vi "Time.vi"() -> ()   [LabVIEW 2025]
panel:
  out "date/time string":string
  out "Waveform Chart":dbl(graph)
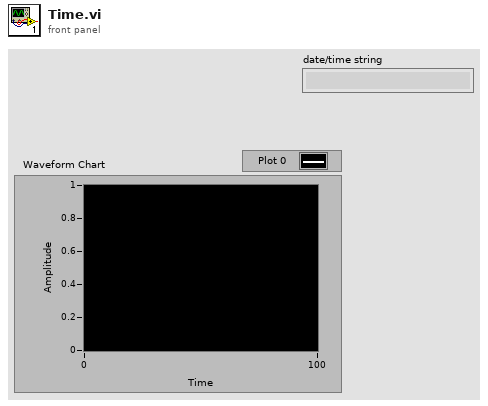
[diagram p1: front panel]
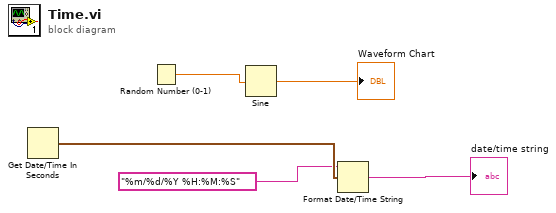
[diagram p0: block diagram]
diagram:
  n1 = Get Date/Time In Seconds() -> (seconds since 1Jan1904=w5:timestamp)
  n2 = Random Number (0-1)() -> (number: 0 to 1=w1:dbl)
  n3 = Sine(x=w1) -> (sin(x)=→"Waveform Chart":dbl)
  n4 = Format Date/Time String(time format string (%c)="%m/%d/%Y %H:%M:%S", seconds (now)=w5) -> (date/time string=→"date/time string":string)  [unwired: 1 in]
